vi "PI Convert Measurement Cluster.vi"(4 "PI Measurement Field Array":T1[](array[typedef])) -> (2 "PI HTML Out":string)   [LabVIEW 2011]
uses:
  server/database/Fields/Field Record.ctl
  server/database/Fields/Field DataTypes.ctl
  server/database/Fields/Field NextItem.ctl
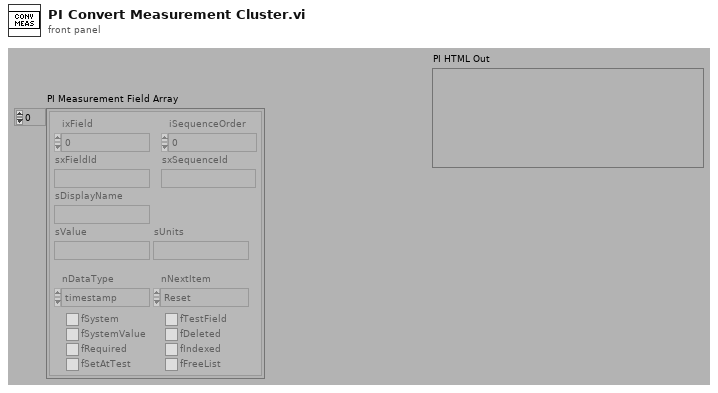
[diagram p1: front panel]
types:
  T1 = typedef "Field Record.ctl" = cluster{"ixField":i32, "iSequenceOrder":i32, "sxFieldId":string, "sxSequenceId":string, "sDisplayName":string, "sValue":string, "sUnits":string, "nDataType":T2, "nNextItem":T3, "fSystem":bool, "fSystemValue":bool, "fRequired":bool, "fSetAtTest":bool, "fTestField":bool, "fDeleted":bool, "fIndexed":bool, "fFreeList":bool}
  T2 = typedef "Field DataTypes.ctl" = enum32{"text", "numeric", "list", "timestamp", "boolean"}
  T3 = typedef "Field NextItem.ctl" = enum32{"Reset", "Retain", "Auto-Increment"}
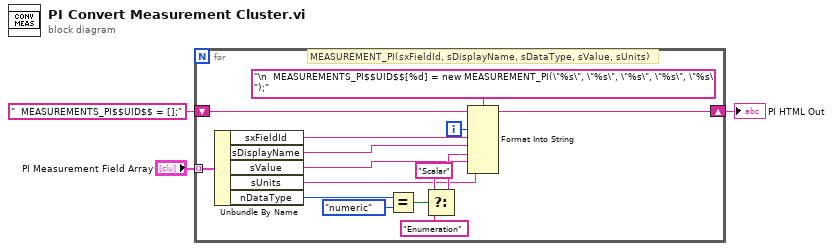
[diagram p0: block diagram]
diagram:
  n1 = for {
    tunnel: "PI Measurement Field Array" -> [w18] mode=indexing
    shift-right: [w15] -> w3
    shift-left: "  MEASUREMENTS_PI$$UID$$ = [];" ("format string") -> [w16]
    i -> [w14]
    # "MEASUREMENT_PI(sxFieldId, sDisplayName, sDataType, sValue, sUnits)"
    n2 = Unbundle By Name(w18) -> ("sxFieldId"=w4:string, "sDisplayName"=w13:string, "sValue"=w7:string, "sUnits"=w6:string, "nDataType"=w5:T2)
    n3 = Equal?(x=w5, y=Field_DataTypes."numeric") -> (x = y?=w8:bool)
    n4 = Select(t="Scalar" ("format string"), s=w8, f="Enumeration" ("format string")) -> (s? t:f=w10:string)
    n5 = Format Into String(format string="\n  MEASUREMENTS_PI$$UID$$[%d] = new MEASUREMENT_PI(\"%s\", \"%s\", \"%s\", \"%s\", \"%s\");", initial string=w16, w14, w4, w13, w10, w7, w6) -> (resulting string=w15:string)  [unwired: 1 in, 1 out]
  }
  "PI HTML Out" <- w3
